vi "CMD_FLEXWRITE.vi"(6 "Gantry Class in":refnum<class "Gantry.lvclass">, 8 "error in (no error)":errorcluster, 10 "Arguments":string[](array[string]), 11 "gScript Interpreter in":refnum<class "gScript Interpreter.lvclass">) -> (0 "error out":errorcluster, 3 "gScript Interpreter out":refnum<class "gScript Interpreter.lvclass">, 4 "Gantry Class out":refnum<class "Gantry.lvclass">)   [LabVIEW 2017, in "gScript Interpreter.lvclass"]
uses:
  gScript Interpreter.lvclass
  Shared Components/Gantry Class/Gantry.lvclass
  Shared Components/FlexWorktable/FlexWorktable.lvclass
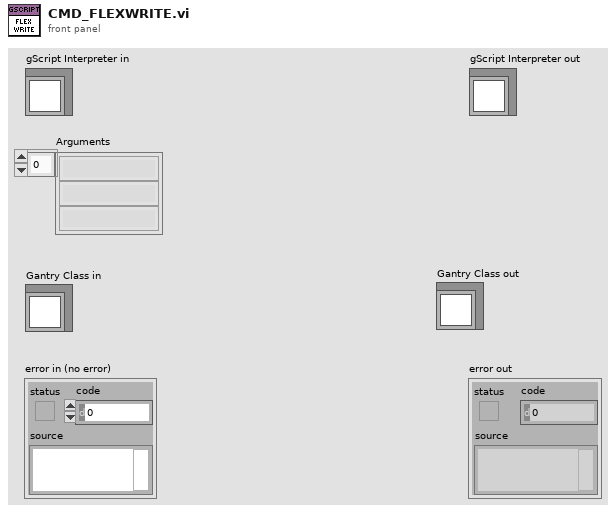
[diagram p1: front panel]
types:
  T1 = typedef "Memory Cell.ctl" = cluster{"type":T2, "x":dbl, "y":dbl, "z":dbl, "w":dbl}
  T2 = typedef "Memory Cell Type Enum.ctl" = enum16{"integer", "float", "vector", "rotation"}
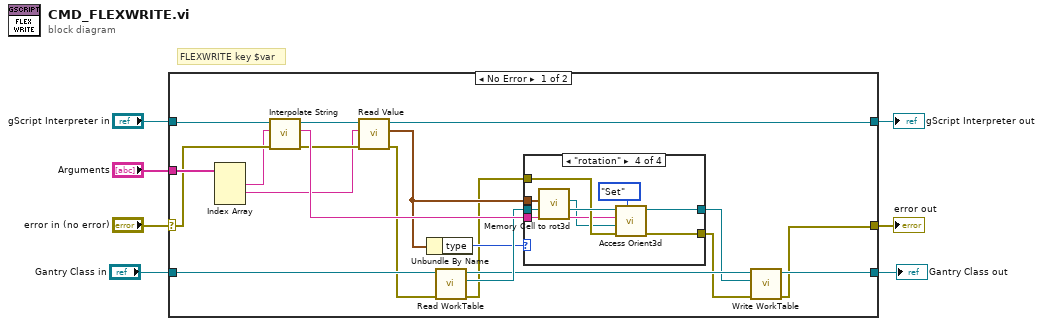
[diagram p0: block diagram]
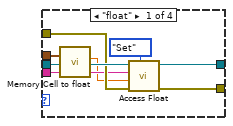
[diagram p2: hidden frame]
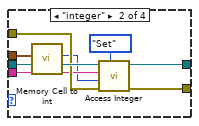
[diagram p3: hidden frame]
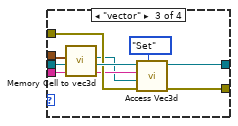
[diagram p4: hidden frame]
diagram:
  # "FLEXWRITE key $var"
  n1 = case shown="No Error" "error in (no error)" {
    selector: "error in (no error)" -> [w25 w62]
    tunnel: [w9 w62] -> w6
    tunnel: [w18 w61] -> w4
    tunnel: "gScript Interpreter in" -> [w26 w61]
    tunnel: "Arguments" -> [w27 _]
    tunnel: "Gantry Class in" -> [w23 w60]
    tunnel: [w10 w60] -> w1
    frame No Error {
      n2 = Index Array(array=w27) -> (element #1=w21:string, element #2=w8:string)  [unwired: 3 in, 1 out]
      n3 = call-dynamic "Interpolate String.vi"("error in (no error)"=w25, "Input String"=w21, "gScript Interpreter in"=w26) -> ("error out"=w19:errorcluster, "Output String"=w24:string, "gScript Interpreter out"=w20:refnum<class "gScript Interpreter.lvclass">)  [unwired: 6 in]
      n4 = call-dynamic "Read Value.vi"("error in (no error)"=w19, "String in"=w8, "gScript Interpreter in"=w20) -> ("error out"=w12:errorcluster, "Memory Cell"=w16:T1, "gScript Interpreter out"=w18:refnum<class "gScript Interpreter.lvclass">)  [unwired: 6 in]
      n5 = Unbundle By Name(w16) -> ("type"=w17:T2)
      n6 = call-dynamic "Read WorkTable.vi"("error in"=w12, "Gantry Class in"=w23) -> ("error out"=w11:errorcluster, "Worktable"=w22:refnum<class "FlexWorktable.lvclass">, "Gantry Class out"=w15:refnum<class "Gantry.lvclass">)  [unwired: 7 in]
      n7 = case shown="\"rotation\"" w17 {
        tunnel: w22 -> [w35 w43 w51 w59]
        tunnel: w11 -> [w34 w42 w49 w58]
        tunnel: [w33 w41 w50 w57] -> w14
        tunnel: w24 -> [w32 w39 w48 w56]
        tunnel: w16 -> [w30 w38 w46 w54]
        tunnel: [w28 w36 w44 w52] -> w13
        frame "float" {
          n8 = call "Memory Cell to float.vi"("Memory Cell"=w30) -> ("float out"=w29:dbl)  [unwired: 10 in]
          n9 = call-dynamic "Access Float.vi"("Get/Set"=enum16{"Get", "Set"}."Set", "error in (no error)"=w34, "Value in"=w29, "Key"=w32, "FlexWorktable in"=w35) -> ("error out"=w33:errorcluster, "FlexWorktable out"=w28:refnum<class "FlexWorktable.lvclass">)  [unwired: 4 in, 1 out]
        }
        frame "integer" {
          n10 = call "Memory Cell to int.vi"("Memory Cell"=w38) -> ("Int out"=w37:i32)  [unwired: 10 in]
          n11 = call-dynamic "Access Integer.vi"("Get/Set"=enum16{"Get", "Set"}."Set", "error in (no error)"=w42, "Value in"=w37, "Key"=w39, "FlexWorktable in"=w43) -> ("error out"=w41:errorcluster, "FlexWorktable out"=w36:refnum<class "FlexWorktable.lvclass">)  [unwired: 4 in, 1 out]
        }
        frame "vector" {
          n12 = call "Memory Cell to vec3d.vi"("Memory Cell"=w46) -> ("Vec3d out"=w45:refnum<class "Vec3d.lvclass">)  [unwired: 10 in]
          n13 = call-dynamic "Access Vec3d.vi"("Get/Set"=enum16{"Get", "Set"}."Set", "error in (no error)"=w49, "Value in"=w45, "Key"=w48, "FlexWorktable in"=w51) -> ("error out"=w50:errorcluster, "FlexWorktable out"=w44:refnum<class "FlexWorktable.lvclass">)  [unwired: 4 in, 1 out]
        }
        frame "rotation" {
          n14 = call "Memory Cell to rot3d.vi"("Memory Cell"=w54) -> ("Orient3d out"=w53:refnum<class "Orient3d.lvclass">)  [unwired: 10 in]
          n15 = call-dynamic "Access Orient3d.vi"("Get/Set"=enum16{"Get", "Set"}."Set", "error in (no error)"=w58, "Value in"=w53, "Key"=w56, "FlexWorktable in"=w59) -> ("error out"=w57:errorcluster, "FlexWorktable out"=w52:refnum<class "FlexWorktable.lvclass">)  [unwired: 4 in, 1 out]
        }
      }
      n16 = call-dynamic "Write WorkTable.vi"("error in (no error)"=w14, "FlexWorktable"=w13, "Gantry Class in"=w15) -> ("error out"=w9:errorcluster, "Gantry Class out"=w10:refnum<class "Gantry.lvclass">)  [unwired: 7 in]
    }
    frame Error {
    }
  }
  "error out" <- w6
  "gScript Interpreter out" <- w4
  "Gantry Class out" <- w1
